vi "ExManualCalibSaveToSpe.vi"() -> ()   [LabVIEW 2010]
panel:
  in  "Full File Name to Write":path=path "C:/Program Files/SIToolKit/LabVIEW/Data Files/CalibHGArgon2.SPE"
  in  "stop":bool
  in  "Finished picking peaks":bool
  out "XY Graph":cluster{dbl[], "Array i32":i32[]}(graph)
  in  "Wavelength 3":dbl=576.96 format="%.2f"
  in  "Pixel 3":dbl=537.0 format="%.2f"
  in  "Wavelength 2":dbl=546.074 format="%.2f"
  in  "Pixel 2":dbl=485.0 format="%.2f"
  in  "Wavelength 1":dbl=435.833 format="%.2f"
  in  "Pixel 1":dbl=301.0 format="%.2f"
  out "error out":errorcluster
  in  "error in (no error)":errorcluster
  in  "FileType":u32=67174400
  in  "Full File Name to Read":path=path "C:/Program Files/SIToolKit/LabVIEW/Data Files/HG-ARGON.TIF"
  # "ExManualCalibSaveToSpe.vi : this example shows how\nto do a manual calibration. First select a file with data in it\nat know peaks (i.e. mercury lamp), then start VI.\nEnter pixel of peak with what wavelength peak should be.\nThis example does three peaks, but more can be used\nif available. Once all pixels and wavelengths have been\nentered then hit the finished button. The displahy will\nnow show a calibrated data with wavelength on the \nx axis. The cursor can be moved around to verify\nthe calibration. Hit stop button when done with calibration.\nUser may want to save calibration points in ascii file so\nthat these values can be used when collecting live data.\nThis example also saves the resulting calibrated data into \nan SPE file."
  # "Input File Type:\nSPE = 67371008\nTIF   = 67174400\nPMI  = 67436544"
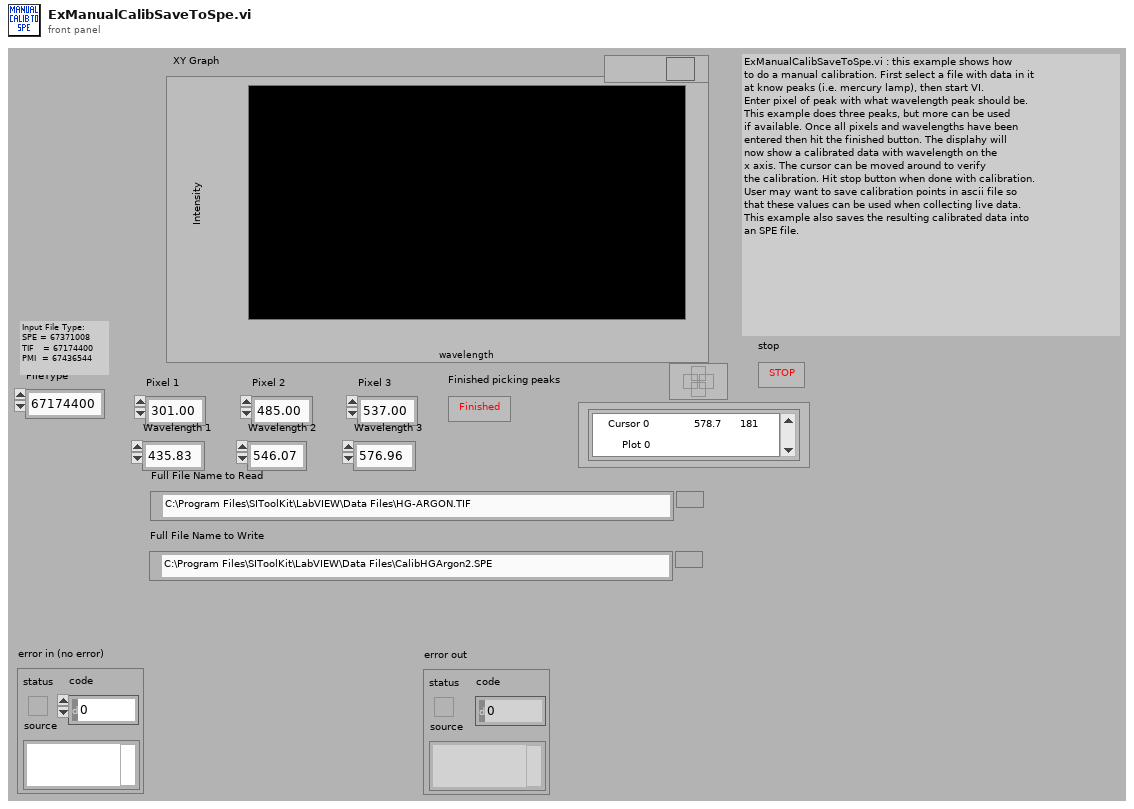
[diagram p1: front panel]
types:
  T1 = cluster{"total pairs":i32, "Order of\npolynominal":i32, "Units in\n4 is  wavelength in nm":i32, "Units out\n4 nm":i32, "Laser line wavelength in nm":dbl}
  T2 = cluster{"Calibrated Array":dbl[], "Array i32":i32[]}
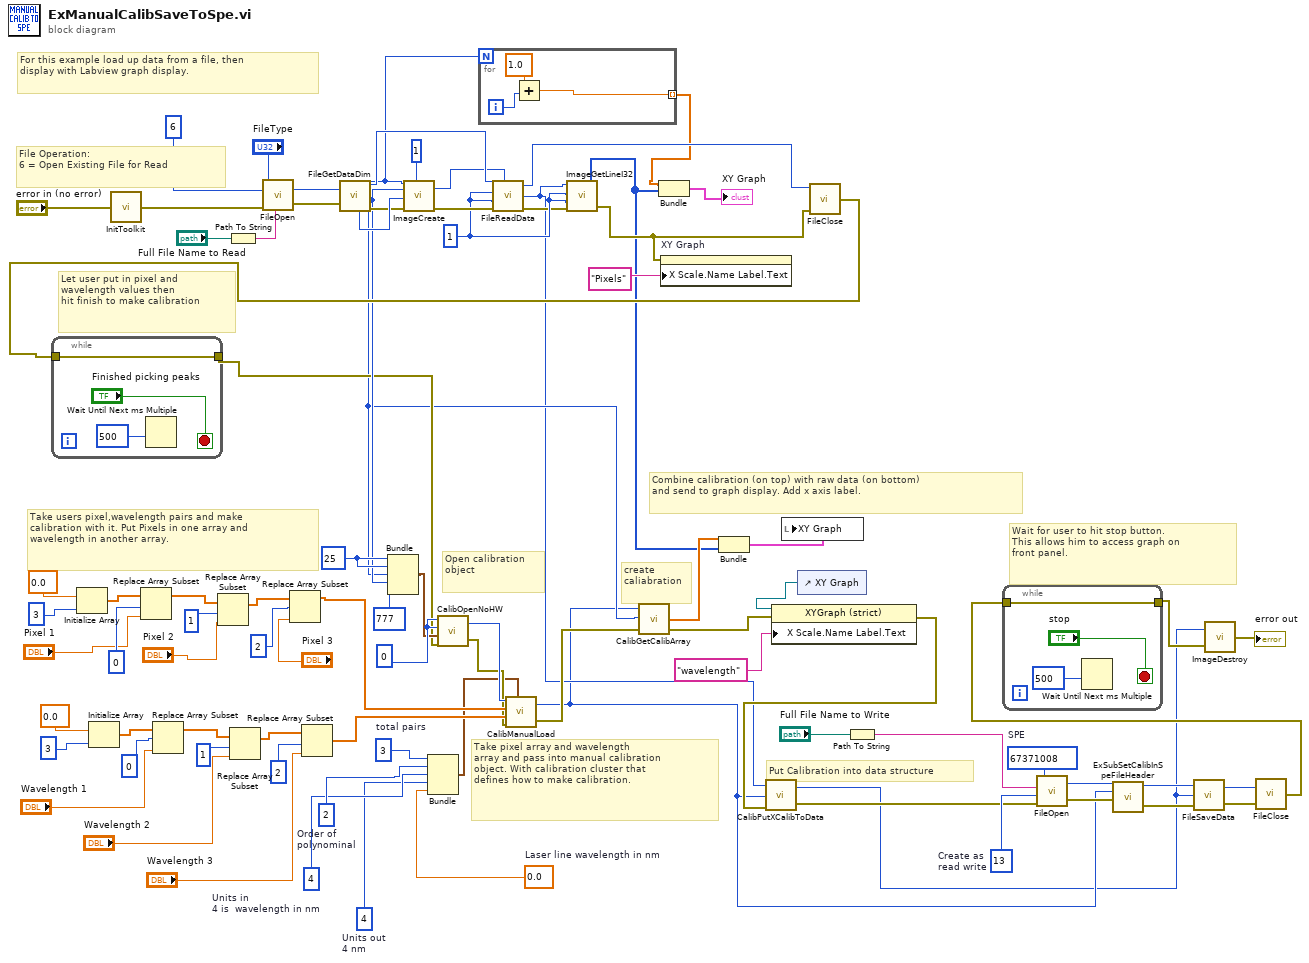
[diagram p0: block diagram]
diagram:
  w16 = 13  # Create as  read write
  w17 = 67371008  # SPE
  w37 = 0.0  # Laser line wavelength in nm
  w38 = 4  # Units out 4 nm
  w39 = 4  # Units in 4 is  wavelength in nm
  w40 = 2  # Order of polynominal
  w41 = 3  # total pairs
  w42 = 0
  w44 = 25
  w73 = 1
  # "Put Calibration into data structure"
  # "Wait for user to hit stop button.\nThis allows him to access graph on\nfront panel."
  # "Combine calibration (on top) with raw data (on bottom) \nand send to graph display. Add x axis label."
  # "create \ncaliabration"
  # "Take pixel array and wavelength \narray and pass into manual calibration \nobject. With calibration cluster that \ndefines how to make calibration."
  # "Open calibration\nobject"
  # "Take users pixel,wavelength pairs and make \ncalibration with it. Put Pixels in one array and\nwavelength in another array."
  # "Let user put in pixel and \nwavelength values then \nhit finish to make calibration"
  # "For this example load up data from a file, then\ndisplay with Labview graph display."
  # "File Operation:\n6 = Open Existing File for Read"
  n1 = Initialize Array(0.0, 3) -> (w61:dbl[])
  n2 = Initialize Array(0.0, 3) -> (w54:dbl[])
  n3 = call <userlib>:"InitToolkit.vi"("error in"="error in (no error)") -> ("error out"=w84:errorcluster)
  n4 = Replace Array Subset(array=w61, new element="Pixel 1", index=0) -> (w60:dbl[])
  n5 = Replace Array Subset(array=w54, new element="Wavelength 1", index=0) -> (w53:dbl[])
  n6 = Replace Array Subset(array=w60, new element="Pixel 2", index=1) -> (w59:dbl[])
  n7 = Path To String(path="Full File Name to Read") -> (string=w78:string)
  n8 = Replace Array Subset(array=w53, new element="Wavelength 2", index=1) -> (w52:dbl[])
  n9 = call <userlib>:"FileOpen.vi"("error in"=w84, "File Operations"=u32 6 ("File Operation"), "FileName"=w78, "File Type"="FileType") -> ("error out"=w82:errorcluster, "File Handle"=w81:u32)
  n10 = Replace Array Subset(array=w59, new element="Pixel 3", index=2) -> (w47:dbl[])
  n11 = Replace Array Subset(array=w52, new element="Wavelength 3", index=2) -> (w48:dbl[])
  n12 = call <userlib>:"FileGetDataDim.vi"("File Handle"=w81, "error in"=w82) -> ("Data Type"=w71:u32, "File Handle"=w76:u32, "X dim"=w26:u32, "Y dim"=w29:u32, "error out"=w70:errorcluster)  [unwired: 1 out]
  n13 = Bundle(w44, w44, "X dim"=w26, "Y dim"=w29, 777) -> (w28:cluster{i32, i32, "X dim":u32, "Y dim":u32, i32})  [unwired: 1 in]
  n14 = call <userlib>:"ImageCreate.vi"("X dimension"=w26, "Y dimension"=w29, "Data Type"=w71, "error in"=w70, "Number Of Frames"=1) -> ("Image Handle"=w75:u32, "error out"=w77:errorcluster)
  n15 = Bundle("total pairs"=w41, "Order of\npolynominal"=w40, "Units in\n4 is  wavelength in nm"=w39, "Units out\n4 nm"=w38, "Laser line wavelength in nm"=w37) -> (w36:T1)  [unwired: 1 in]
  n16 = for {
    N: w26 -> [_]
    tunnel: [w87] -> w69 mode=indexing
    i -> [w88]
    n17 = Add(x=1.0, y=w88) -> (x+y=w87:dbl)
  }
  n18 = call <userlib>:"FileReadData.vi"("File Handle"=w76, "Start Frame"=w73, "End Frame"=w73, "error in"=w77, "Image Handle"=w75) -> ("File Handle"=w74:u32, "Image Handle"=w3:u32, "error out"=w72:errorcluster)
  n19 = call <userlib>:"ImageGetLineI32.vi"("error in"=w72, "Z Position"=w73, "Y Position"=w73, "Data Handle"=w3) -> ("error out"=w66:errorcluster, "Array i32"=w20:i32[])  [unwired: 1 out]
  n20 = Bundle(w69, "Array i32"=w20) -> (→"XY Graph":cluster{dbl[], "Array i32":i32[]})  [unwired: 1 in]
  n21 = property on="XY Graph" class="XYGraph (strict)"(error in=w66, "X Scale.Name Label.Text"="Pixels") -> ()  [unwired: 1 in, 2 out]
  n22 = control-ref of="XY Graph"() -> (w23:refnum<vi>)
  n23 = call <userlib>:"FileClose.vi"("error in"=w66, "File Handle"=w74) -> ("error out"=w65:errorcluster)
  n24 = while {
    tunnel: w65 -> [w91]
    tunnel: [w91] -> w27
    stop <- "Finished picking peaks" stop-if-true
    n25 = Wait Until Next ms Multiple(millisecond multiple=500) -> ()  [unwired: 1 out]
  }
  n26 = call <userlib>:"CalibOpenNoHW.vi"("error in"=w27, "Data Info"=w28, "Calibration Type"=w42, "Calibration Device ID"=w42) -> ("error out"=w45:errorcluster, "Calibration Handle"=w46:u32)
  n27 = call <userlib>:"CalibManualLoad.vi"("Calibration Handle"=w46, "Pixel Array"=w47, "Wavelength Array"=w48, "error in (no error)"=w45, "Calibration Values"=w36) -> ("Calibration Handle"=w2:u32, "error out"=w11:errorcluster)
  n28 = call <userlib>:"CalibGetCalibArray.vi"("error in"=w11, "Array Size"=w26, "Calibration Handle"=w2) -> ("error out"=w24:errorcluster, "Calibrated Array"=w21:dbl[])  [unwired: 1 out]
  n29 = Bundle("Calibrated Array"=w21, "Array i32"=w20) -> (w25:T2)  [unwired: 1 in]
  n30 = property on="Property Node" class="XYGraph (strict)"(reference=w23, error in=w24, "X Scale.Name Label.Text"="wavelength") -> (error out=w12:errorcluster)  [unwired: 1 out]
  n31 = call <userlib>:"CalibPutXCalibToData.vi"("error in (no error)"=w12, "Calibration Handle"=w2, "Data Handle"=w3) -> ("error out"=w15:errorcluster, "Data Handle"=w1:u32)
  n32 = local write "XY Graph"(w25) -> ()
  n33 = Path To String(path="Full File Name to Write") -> (string=w18:string)
  n34 = call <userlib>:"FileOpen.vi"("error in"=w15, "File Operations"=w16, "FileName"=w18, "File Type"=w17) -> ("error out"=w6:errorcluster, "File Handle"=w7:u32)
  n35 = call "ExSubSetCalibInSpeFileHeader.vi"("error in (no error)"=w6, "Calibration Handle"=w2, "File Handle"=w7) -> ("error out"=w4:errorcluster, "File Handle"=w5:u32)  [unwired: 1 out]
  n36 = call <userlib>:"FileSaveData.vi"("error in"=w4, "Image Handle"=w1, "File Handle"=w5) -> ("error out"=w14:errorcluster, "File Handle"=w13:u32)
  n37 = call <userlib>:"FileClose.vi"("error in"=w14, "File Handle"=w13) -> ("error out"=w10:errorcluster)
  n38 = while {
    tunnel: w10 -> [w93]
    tunnel: [w93] -> w9
    stop <- "stop" stop-if-true
    n39 = Wait Until Next ms Multiple(millisecond multiple=500) -> ()  [unwired: 1 out]
  }
  n40 = call <userlib>:"ImageDestroy.vi"("error in"=w9, "Data handle"=w1) -> ("error out"=→"error out":errorcluster)
